vi "DHE_set_geom.vi"(0 "fd":i32, 1 "ypredata":i32, 2 "ypostdata":i32, 5 "xpredata":i32, 7 "xpostdata":i32, 9 "xdata":i32, 11 "error in (no error)":errorcluster, 12 "ydata":i32) -> (4 "fd out":i32, 8 "return value":i32, 15 "error out":errorcluster)   [LabVIEW 2016]
doc: "This VI closes the I/O interface with the instrument."
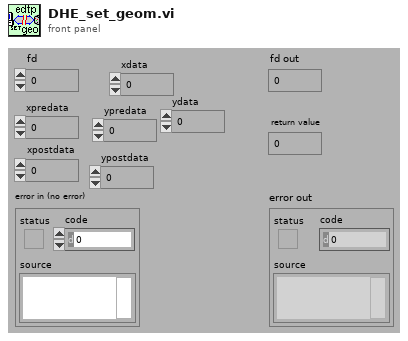
[diagram p1: front panel]
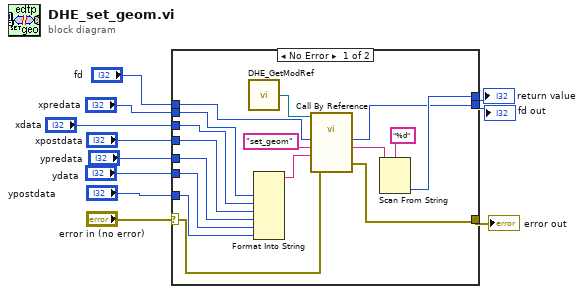
[diagram p0: block diagram]
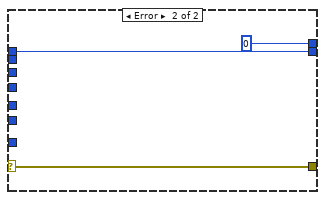
[diagram p2: hidden frame]
diagram:
  n1 = case shown="No Error" "error in (no error)" {
    selector: "error in (no error)" -> [w15 w28]
    tunnel: "fd" -> [w19 w30]
    tunnel: [w21 0] -> w10
    tunnel: [w22 w28] -> w9
    tunnel: "xpredata" -> [w18 _]
    tunnel: "xpostdata" -> [w16 _]
    tunnel: [w20 w30] -> w6
    tunnel: "ypredata" -> [w14 _]
    tunnel: "ypostdata" -> [w12 _]
    tunnel: "ydata" -> [w13 _]
    tunnel: "xdata" -> [w17 _]
    frame No Error {
      n2 = call "DHE_GetModRef.vi"() -> ("DHE_ModRef"=w27:refnum<vi>)  [unwired: 9 out]
      n3 = Format Into String(w18, w17, w16, w14, w13, w12) -> (resulting string=w23:string)  [unwired: 3 in, 1 out]
      n4 = call-by-ref "?"(reference=w27, "error in (no error)"=w15, "arguments"=w23, "function"="set_geom", "fd in"=w19) -> ("error out"=w22:errorcluster, "str result"=w25:string, "fd out"=w20:i32)  [unwired: 5 in, 3 out]
      n5 = Scan From String(format string="%d", input string=w25) -> (output 1=w21:i32)  [unwired: 2 in, 4 out]
    }
    frame Error {
    }
  }
  "error out" <- w9
  "return value" <- w10
  "fd out" <- w6
